vi "Configure Device.vi"(8 "error in (no error)":errorcluster, 10 "Max beams":dbl, 11 "Toggle 8 in":refnum<class "Toggle 8.lvclass">) -> (0 "error out":errorcluster, 3 "Toggle 8 out":refnum<class "Toggle 8.lvclass">)   [LabVIEW 2020, in "Toggle 8.lvclass"]
doc: "Interface for configuring the device for testing"
uses:
  Toggle 8.lvclass
  C:/Sandbox/Git_Sandbox/WiSpry Test Framework source code (LV20)/WiSpry Test Framework/Devices/Device.lvclass
  Controls/Test Sequence.ctl
  Controls/Register to Write.ctl
  PIC-device/PIC-Device.lvclass
panel:
  in  "Custom initialization":T1={"Enable"=FALSE, "User init values"="074000,\n074101,\nV1,\n07427F,\n07437F,\n074B01,\n074C20,\n074080,\nd200,\n074C31,\nd200"}
  in  "Loop order":bool
  in  "Pre-measurement cycling":cluster{"Cycle":bool, "Number of cycles":u32}={"Cycle"=FALSE, "Number of cycles"=2000}
  in  "CPV":T2(ring)=enum."CP 45V"
  in  "CP values":string="44" caption="CP Voltage"
  in  "USID":bool=TRUE
  in  "Read Info":bool
  in  "Clear all":bool
  in  "Beams Sequentially":bool
  in  "All Beams Individually":bool
  in  "OK Button":bool
  in  "Control individual beams":bool
  in  "REG2-3":u8[][](array[numeric])=[[0, 0], [8, 0], [0, 8]] format="%x"
  in  "Capa values":string="0:31/1" caption="OTP Capacitance value (dec)"
  out "Selected CP Voltages":T3(array[ring])=[enum."CP 44V"]
  # "Cycling counter resets \nwhen device information \nis changed."
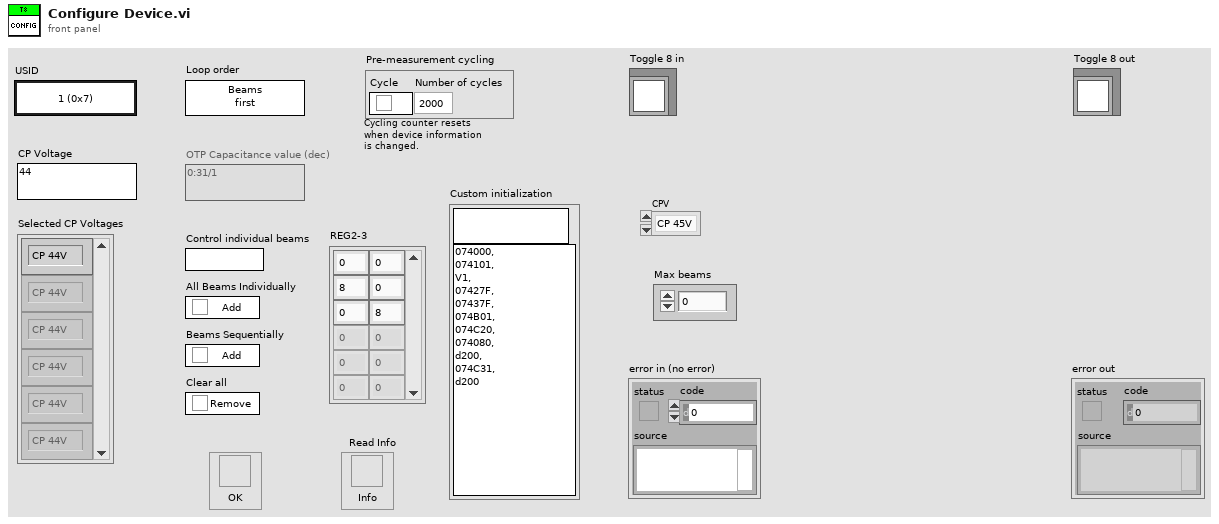
[diagram p1: front panel]
types:
  T1 = cluster{"Enable":bool, "User init values":string}
  T2 = enum16{"CP 24V", "CP 26V", "CP 28V", "CP 30V", "CP 31V", "CP 32V", "CP 33V", "CP 34V", "CP 35V", "CP 36V", "CP 37V", "CP 38V", "CP 39V", "CP 40V", "CP 41V", "CP 42V", "CP 43V", "CP 44V", "CP 45V", "CP 46V", "CP 47V", "CP 48V", "CP 49V", "CP 50V", "CP 51V", "CP 52V", "CP 53V", "CP 54V", "CP 56V", "CP 58V", "CP 60V", "CP 62V"}
  T3 = enum16{"CP 24V", "CP 26V", "CP 28V", "CP 30V", "CP 31V", "CP 32V", "CP 33V", "CP 34V", "CP 35V", "CP 36V", "CP 37V", "CP 38V", "CP 39V", "CP 40V", "CP 41V", "CP 42V", "CP 43V", "CP 44V", "CP 45V", "CP 46V", "CP 47V", "CP 48V", "CP 49V", "CP 50V", "CP 51V", "CP 52V", "CP 53V", "CP 54V", "CP 56V", "CP 58V", "CP 60V", "CP 62V"}[]
  T4 = cluster{"CP values":refnum<vi>, "CP Voltage":refnum<vi>, "Control individual beams":refnum<vi>, "REG2-3":refnum<vi>, "Capa values":refnum<vi>, "Custom init":refnum<vi>, "User init":refnum<vi>}
  T5 = typedef "Toggle 8.lvclass/Test Sequence.ctl" = cluster{"CP values":string, "Charge Pump values":enum16{"CP 24V", "CP 26V", "CP 28V", "CP 30V", "CP 31V", "CP 32V", "CP 33V", "CP 34V", "CP 35V", "CP 36V", "CP 37V", "CP 38V", "CP 39V", "CP 40V", "CP 41V", "CP 42V", "CP 43V", "CP 44V", "CP 45V", "CP 46V", "CP 47V", "CP 48V", "CP 49V", "CP 50V", "CP 51V", "CP 52V", "CP 53V", "CP 54V", "CP 56V", "CP 58V", "CP 60V", "CP 62V"}[], "Charge Pump":T6[], "Control individual beams":bool, "OTP/beam values":dbl[], "Capa settings":T6[], "OTP Values string":string}
  T6 = typedef "PIC-Device.lvclass/Register to Write.ctl" = cluster{"Register":u32, "Value":u32, "Dev Address":u32, "Physical Adress":u32}
  T7 = cluster{"Cycle":bool, "Number of cycles":u32, "Cycles Executed":u32}
  T8 = enum8{"Enabled", "Disabled", "Disabled and Grayed Out"}
  T9 = typedef "Device.lvclass/Device Information Cluster.ctl" = cluster{"Device Info":string[][], "Default Values":T6[], "Fetched info":string[][]}
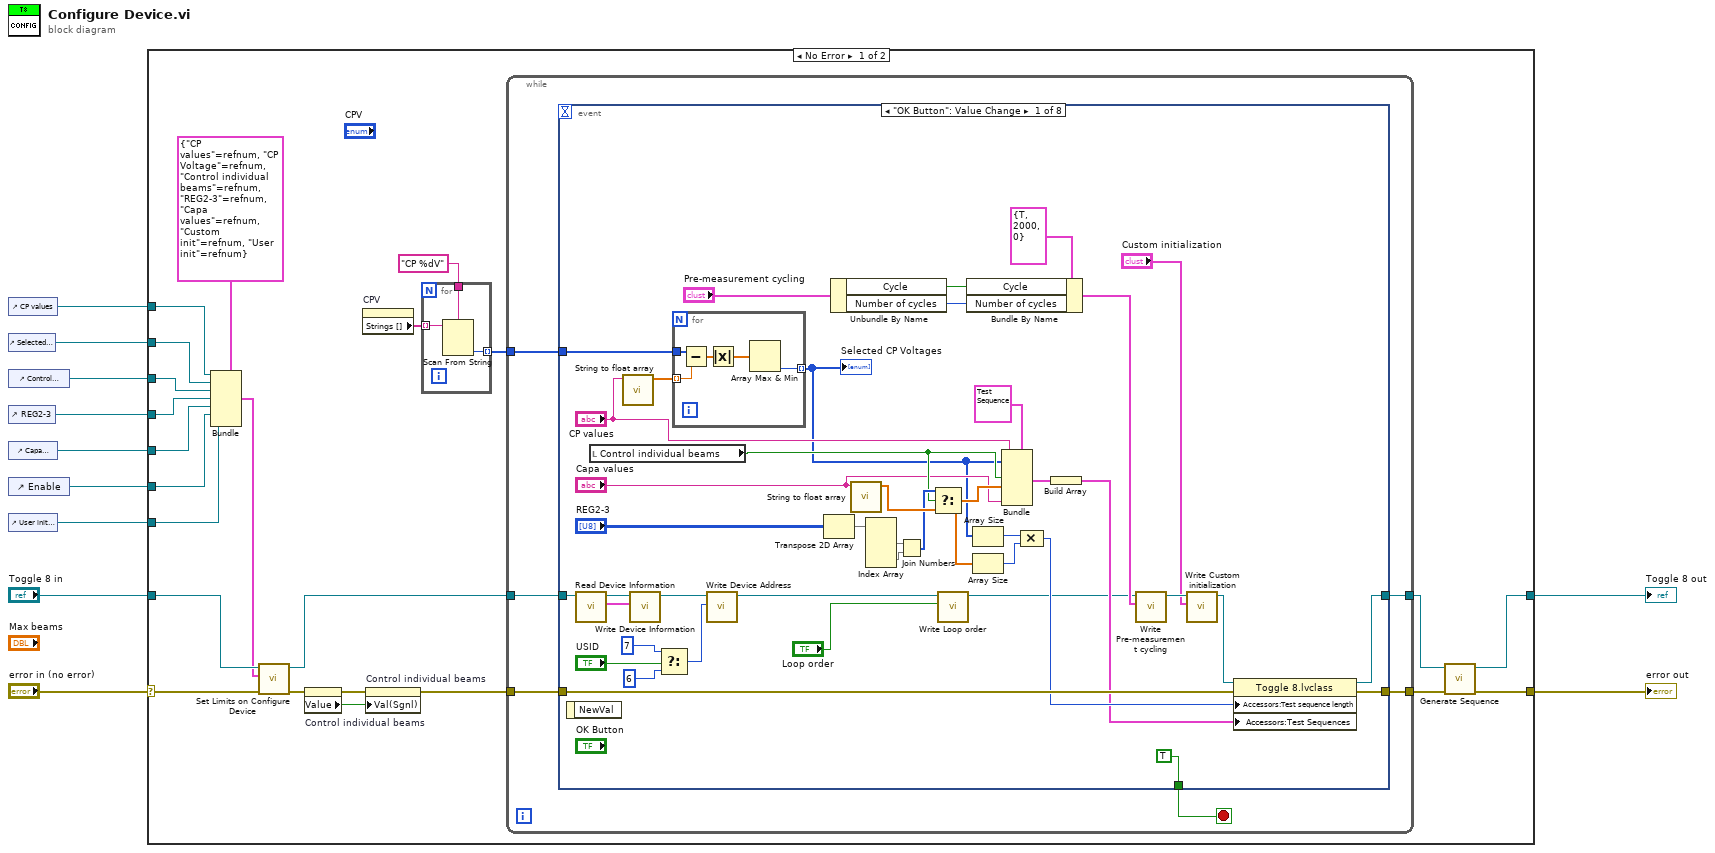
[diagram p0: block diagram]
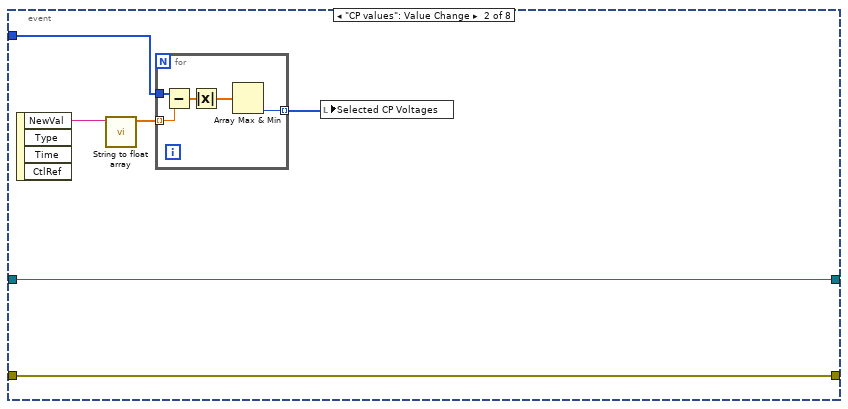
[diagram p2: hidden frame]
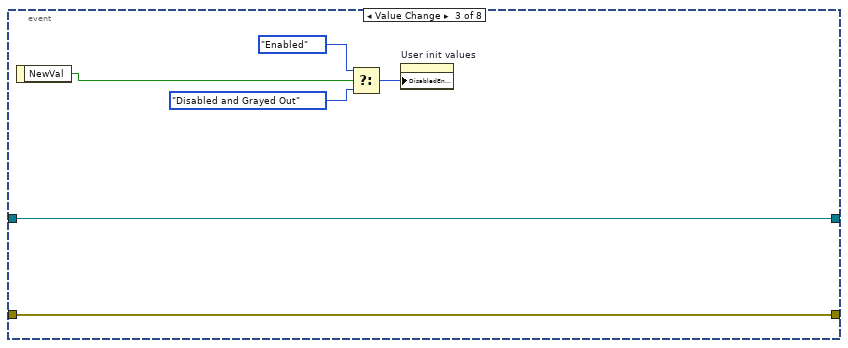
[diagram p3: hidden frame]
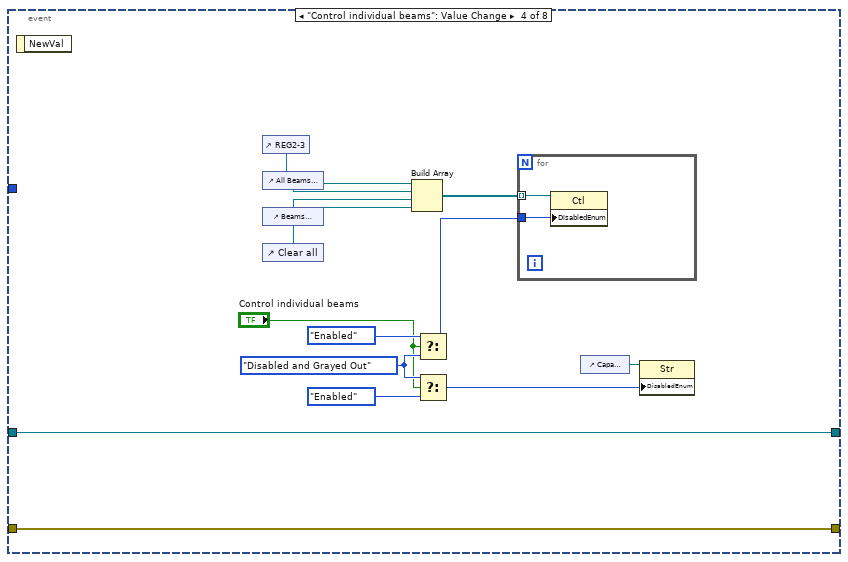
[diagram p4: hidden frame]
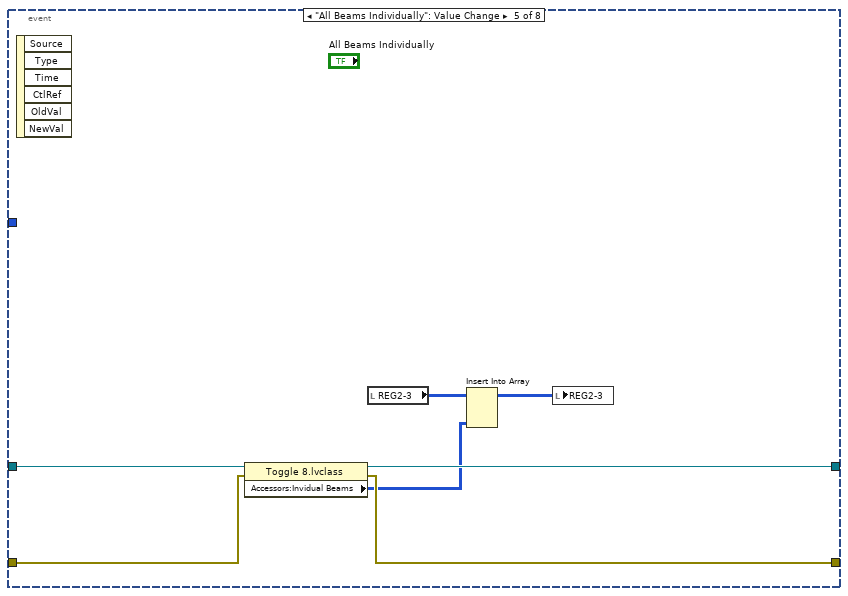
[diagram p5: hidden frame]
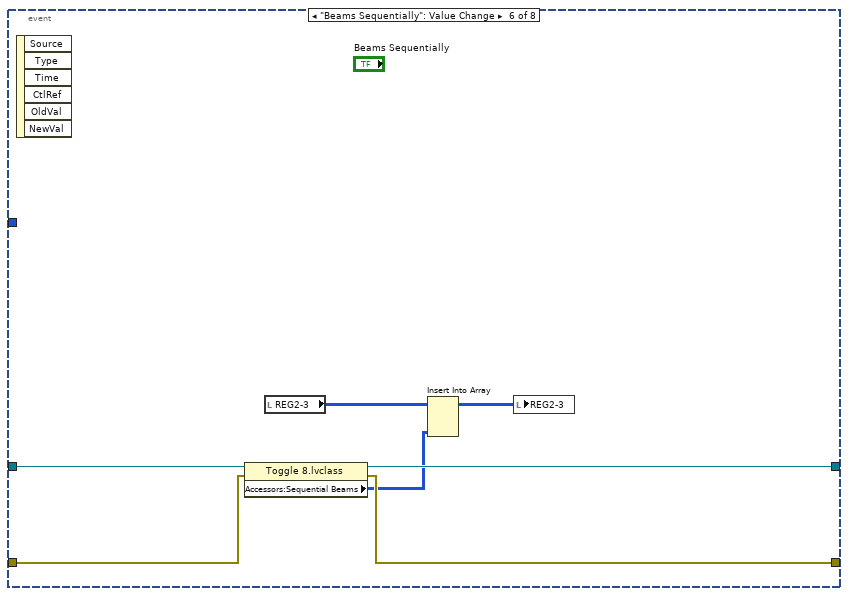
[diagram p6: hidden frame]
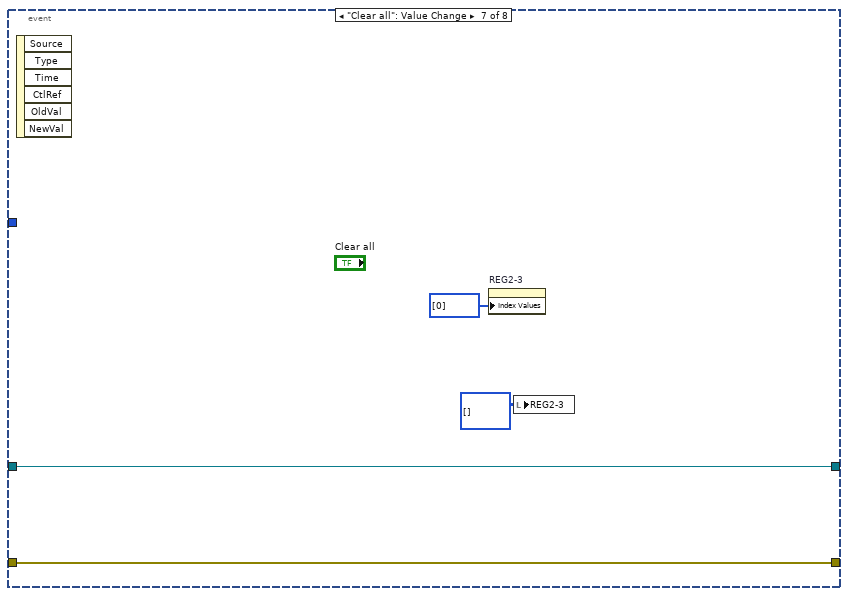
[diagram p7: hidden frame]
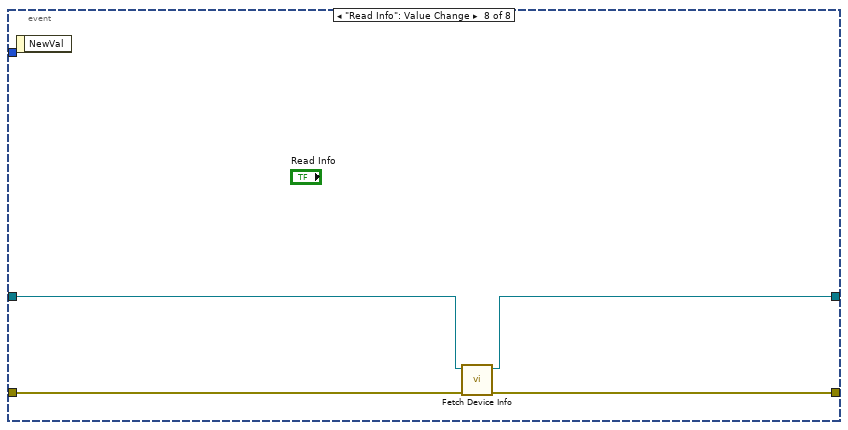
[diagram p8: hidden frame]
diagram:
  n1 = control-ref of="CP values"() -> (w3:refnum<vi>)
  n2 = control-ref of="Selected CP Voltages"() -> (w4:refnum<vi>)
  n3 = control-ref of="Control individual beams"() -> (w5:refnum<vi>)
  n4 = control-ref of="REG2-3"() -> (w6:refnum<vi>)
  n5 = control-ref of="Capa values"() -> (w7:refnum<vi>)
  n6 = control-ref of="Enable"() -> (w2:refnum<vi>)
  n7 = control-ref of="User init values"() -> (w1:refnum<vi>)
  n8 = case shown="No Error" "error in (no error)" {
    selector: "error in (no error)" -> [w20 w147]
    tunnel: [w30 w147] -> w10
    tunnel: "Toggle 8 in" -> [w26 w146]
    tunnel: [w28 w146] -> w8
    tunnel: w7 -> [w24 _]
    tunnel: w6 -> [w23 _]
    tunnel: w5 -> [w22 _]
    tunnel: w4 -> [w21 _]
    tunnel: w3 -> [w17 _]
    tunnel: w2 -> [w13 _]
    tunnel: w1 -> [w12 _]
    frame No Error {
      n9 = Bundle(cluster=T4 {"CP values"=refnum, "CP Voltage"=refnum, "Control individual beams"=refnum, "REG2-3"=refnum, "Capa values"=refnum, "Custom init"=refnum, "User init"=refnum} ("Toggle8 controls cluster"), "CP values"=w17, "CP Voltage"=w21, "Control individual beams"=w22, "REG2-3"=w23, "Capa values"=w24, "Custom init"=w13, "User init"=w12) -> (w18:T4)
      n10 = call "Set Limits on Configure Device.vi"("error in (no error)"=w20, "Toggle8 controls cluster"=w18, "Toggle 8 in"=w26) -> ("error out"=w19:errorcluster, "Toggle 8 out"=w25:refnum<class "Toggle 8.lvclass">)  [unwired: 7 in]
      n11 = property on="Control individual beams" class="Bool (strict)"(error in=w19) -> (error out=w33:errorcluster, "Value"=w34:bool)  [unwired: 1 in, 1 out]
      n12 = property on="CPV" class="Enum (strict)"() -> ("Strings []"=w16:string[])  [unwired: 2 in, 2 out]
      n13 = property on="Control individual beams" class="Bool (strict)"(error in=w33, "Val(Sgnl)"=w34) -> (error out=w32:errorcluster)  [unwired: 1 in, 1 out]
      n14 = for {
        tunnel: w16 -> [w36] mode=indexing
        tunnel: "CP %dV" ("format string") -> [w37]
        tunnel: [w35] -> w14 mode=indexing
        n15 = Scan From String(format string=w37, input string=w36) -> (output 1=w35:i32)  [unwired: 3 in, 3 out]
      }
      n16 = while {
        tunnel: w25 -> [w43]
        tunnel: [w41] -> w29
        tunnel: w32 -> [w40]
        tunnel: [w39] -> w31
        tunnel: w14 -> [w38]
        stop <- w42 stop-if-true
        n17 = event shown="[0] \"OK Button\": Value Change" {
          selector: _ -> [_ _ _ _ _ _ _ _]
          dyn-events: _ -> [_ _ _ _ _ _ _ _]
          timeout: _ -> [_ _ _ _ _ _ _ _]
          tunnel: w43 -> [w69 w92 w103 w108 w130 w137 w141 w144]
          tunnel: [TRUE _ _ _ _ _ _ _] -> w42
          tunnel: [w83 w92 w103 w108 w129 w136 w141 w142] -> w41
          tunnel: w40 -> [w79 w91 w102 w109 w128 w135 w140 w145]
          tunnel: [w78 w91 w102 w109 w127 w134 w140 w143] -> w39
          tunnel: w38 -> [w52 w94 _ _ _ _ _ _]
          event "OK Button": Value Change {
            n18 = event-data() -> ()  [unwired: 1 in, 1 out]
            n19 = call-dynamic "Read Device Information.vi"("Device in"=w69) -> ("Device Info"=w68:T9[], "Device out"=w70:refnum<class "Toggle 8.lvclass">)  [unwired: 8 in, 1 out]
            n20 = local read "Control individual beams"() -> (w71:bool)
            n21 = call "String to float array.vi"("String"="CP values") -> ("Array - Numeric"=w53:dbl[])  [unwired: 9 in, 1 out]
            n22 = call-dynamic "Write Device Information.vi"("Device Info"=w68, "Device in"=w70) -> ("Device out"=w65:refnum<class "Toggle 8.lvclass">)  [unwired: 8 in, 1 out]
            n23 = Select(t=u8 7 ("Device Address"), s="USID", f=u8 6 ("Device Address")) -> (s? t:f=w61:u8)
            n24 = for {
              tunnel: w53 -> [w89] mode=indexing
              tunnel: w52 -> [w90]
              tunnel: [w88] -> w51 mode=indexing
              n25 = Subtract(x=w90, y=w89) -> (x-y=w87:dbl[])
              n26 = Absolute Value(x=w87) -> (abs(x)=w86:dbl[])
              n27 = Array Max & Min(array=w86) -> (min index (indices)=w88:i32)  [unwired: 3 out]
            }
            "Selected CP Voltages" <- w51
            n28 = call-dynamic "Write Device Address.vi"("Device Address"=w61, "PIC-Device in"=w65) -> ("PIC-Device out"=w49:refnum<class "Toggle 8.lvclass">)  [unwired: 9 in]
            n29 = Transpose 2D Array(2D array="REG2-3") -> (transposed array=w81:u8[][])
            n30 = Unbundle By Name("Pre-measurement cycling") -> ("Cycle"=w58:bool, "Number of cycles"=w59:u32)
            n31 = call "String to float array.vi"("String"="Capa values") -> ("Array - Numeric"=w82:dbl[])  [unwired: 9 in, 1 out]
            n32 = Index Array(array=w81) -> (element #1=w77:u8[], element #2=w76:u8[])  [unwired: 4 in]
            n33 = Join Numbers(hi=w77, lo=w76) -> ((hi.lo)=w75:u16[])
            n34 = Select(t=w75, s=w71, f=w82) -> (s? t:f=w74:dbl[])
            n35 = call-dynamic "Write Loop order.vi"("Loop order"="Loop order", "Toggle 8 in"=w49) -> ("Toggle 8 out"=w48:refnum<class "Toggle 8.lvclass">)  [unwired: 9 in]
            n36 = Bundle By Name(cluster=T7 {"Cycle"=TRUE, "Number of cycles"=2000, "Cycles Executed"=0} ("Pre-measurement cycling"), "Cycle"=w58, "Number of cycles"=w59) -> (w57:T7)
            n37 = Array Size(array=w51) -> (size(s)=w73:i32)
            n38 = Array Size(array=w74) -> (size(s)=w72:i32)
            n39 = Bundle(cluster=T5 {"CP values"="44", "Charge Pump values"=[], "Charge Pump"=[{"Register"=0, "Value"=0, "Dev Address"=7, "Physical Adress"=0}, {"Register"=0, "Value"=128, "Dev Address"=7, "Physical Adress"=0}], "Control individual beams"=FALSE, "OTP/beam values"=[], "Capa settings"=[{"Register"=0, "Value"=0, "Dev Address"=7, "Physical Adress"=0}, {"Register"=0, "Value"=128, "Dev Address"=7, "Physical Adress"=0}], "OTP Values string"=""} ("Test Sequence"), "CP values"="CP values", "Charge Pump values"=w51, "Control individual beams"=w71, "OTP/beam values"=w74, "OTP Values string"="Capa values") -> (w84:T5)  [unwired: 2 in]
            n40 = Compound Arithmetic op=MULTIPLY(w73, w72) -> (w67:i32)
            n41 = Build Array(w84) -> (w55:T5[])
            n42 = call-dynamic "Write Pre-measurement cycling.vi"("Pre-measurement cycling"=w57, "PIC-Device in"=w48) -> ("PIC-Device out"=w46:refnum<class "Toggle 8.lvclass">)  [unwired: 9 in]
            n43 = call-dynamic "Write Custom initialization.vi"("Custom initialization"="Custom initialization", "Toggle 8 in"=w46) -> ("Toggle 8 out"=w45:refnum<class "Toggle 8.lvclass">)  [unwired: 9 in]
            n44 = property class="Toggle 8.lvclass"(reference=w45, error in=w79, "Accessors:Test sequence length"=w67, "Accessors:Test Sequences"=w55) -> (reference out=w83:refnum<class "Toggle 8.lvclass">, error out=w78:errorcluster)
          }
          event "CP values": Value Change {
            n45 = event-data() -> ("NewVal"=w95:string)  [unwired: 1 in, 3 out]
            n46 = call "String to float array.vi"("String"=w95) -> ("Array - Numeric"=w96:dbl[])  [unwired: 9 in, 1 out]
            n47 = for {
              tunnel: w96 -> [w100] mode=indexing
              tunnel: w94 -> [w101]
              tunnel: [w99] -> w93 mode=indexing
              n48 = Subtract(x=w101, y=w100) -> (x-y=w98:dbl[])
              n49 = Absolute Value(x=w98) -> (abs(x)=w97:dbl[])
              n50 = Array Max & Min(array=w97) -> (min index (indices)=w99:i32)  [unwired: 3 out]
            }
            n51 = local write "Selected CP Voltages"(w93) -> ()
          }
          event "Custom initialization.Enable": Value Change {
            n52 = event-data() -> ("NewVal"=w104:bool)  [unwired: 1 in]
            n53 = Select(t=T8."Enabled" ("Disabled"), s=w104, f=T8."Disabled and Grayed Out" ("Disabled")) -> (s? t:f=w105:T8)
            n54 = property on="User init values" class="Str"("DisabledEnum"=w105) -> ()  [unwired: 2 in, 2 out]
          }
          event "Control individual beams": Value Change {
            w114 = T8."Disabled and Grayed Out" ("Disabled")
            n55 = event-data() -> ()  [unwired: 1 in, 1 out]
            n56 = control-ref of="REG2-3"() -> (w121:refnum<vi>)
            n57 = control-ref of="All Beams Individually"() -> (w120:refnum<vi>)
            n58 = control-ref of="Beams Sequentially"() -> (w119:refnum<vi>)
            n59 = control-ref of="Clear all"() -> (w118:refnum<vi>)
            n60 = Build Array(w121, w120, w119, w118) -> (w117:refnum<vi>[])
            n61 = Select(t=T8."Enabled" ("Disabled"), s="Control individual beams", f=w114) -> (s? t:f=w111:T8)
            n62 = Select(t=w114, s="Control individual beams", f=T8."Enabled" ("Disabled")) -> (s? t:f=w110:T8)
            n63 = for {
              tunnel: w117 -> [w123] mode=indexing
              tunnel: w111 -> [w122]
              n64 = property class="Ctl"(reference=w123, "DisabledEnum"=w122) -> ()  [unwired: 1 in, 2 out]
            }
            n65 = control-ref of="Capa values"() -> (w116:refnum<vi>)
            n66 = property class="Str"(reference=w116, "DisabledEnum"=w110) -> ()  [unwired: 1 in, 2 out]
          }
          event "All Beams Individually": Value Change {
            n67 = event-data() -> ()  [unwired: 1 in, 6 out]
            n68 = property class="Toggle 8.lvclass"(reference=w130, error in=w128) -> (reference out=w129:refnum<class "Toggle 8.lvclass">, error out=w127:errorcluster, "Accessors:Invidual Beams"=w125:u8[][])
            n69 = local read "REG2-3"() -> (w126:u8[][])
            n70 = Insert Into Array(array=w126, new element=w125) -> (w124:u8[][])  [unwired: 2 in]
            n71 = local write "REG2-3"(w124) -> ()
          }
          event "Beams Sequentially": Value Change {
            n72 = event-data() -> ()  [unwired: 1 in, 6 out]
            n73 = property class="Toggle 8.lvclass"(reference=w137, error in=w135) -> (reference out=w136:refnum<class "Toggle 8.lvclass">, error out=w134:errorcluster, "Accessors:Sequential Beams"=w131:u8[][])
            n74 = local read "REG2-3"() -> (w133:u8[][])
            n75 = Insert Into Array(array=w133, new element=w131) -> (w132:u8[][])  [unwired: 2 in]
            n76 = local write "REG2-3"(w132) -> ()
          }
          event "Clear all": Value Change {
            n77 = event-data() -> ()  [unwired: 1 in, 6 out]
            n78 = property on="REG2-3" class="Arr (strict)"("Index Values"=u32[] [0]) -> ()  [unwired: 2 in, 2 out]
            n79 = local write "REG2-3"(u8[][] [] ("REG2-3")) -> ()
          }
          event "Read Info": Value Change {
            n80 = event-data() -> ()  [unwired: 1 in, 1 out]
            n81 = call-dynamic "Fetch Device Info.vi"("error in (no error)"=w145, "Toggle 8 in"=w144) -> ("error out"=w143:errorcluster, "Toggle 8 out"=w142:refnum<class "Toggle 8.lvclass">)  [unwired: 7 in, 1 out]
          }
        }
      }
      n82 = call-dynamic "Generate Sequence.vi"("error in (no error)"=w31, "Toggle 8 in"=w29) -> ("error out"=w30:errorcluster, "Toggle 8 out"=w28:refnum<class "Toggle 8.lvclass">)  [unwired: 8 in]
    }
    frame Error {
    }
  }
  "error out" <- w10
  "Toggle 8 out" <- w8
